vi "Climb Ramp.vi"(10 "Climb":bool, 11 "Plummet":bool) -> ()   [LabVIEW 2016]
uses:
  <vilib>/addons/control/pid/pid.llb/PID Control Input Filter (DBL).vi
  <vilib>/addons/control/pid/NI_PID_pid.lvlib
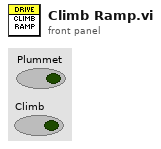
[diagram p1: front panel]
types:
  T1 = typedef "WPI_MotorControlDeviceRef.ctl" = cluster{"DeviceStatus":errorcluster, "Type":T2, "PWM":cluster{"PWM Channel":T3, "DeadBand":T4}, "CAN":cluster{"Device Number":u8, "SetOutput VI Ref":variant, "GetOutput VI Ref":variant, "Enable VI Ref":variant, "Disable VI Ref":variant, "Data":variant}, "Invert":bool}
  T2 = typedef "WPI_MotorControlType.ctl" = enum16{"PWM", "CAN"}
  T3 = typedef "FPGA_DIOPWMChannel.ctl" = enum8{"PWM 0", "PWM 1", "PWM 2", "PWM 3", "PWM 4", "PWM 5", "PWM 6", "PWM 7", "PWM 8", "PWM 9", "PWM MXP 0", "PWM MXP 1", "PWM MXP 2", "PWM MXP 3", "PWM MXP 4", "PWM MXP 5", "PWM MXP 6", "PWM MXP 7", "PWM MXP 8", "PWM MXP 9", "Invalid"}
  T4 = typedef "WPI_PWMDeadband.ctl" = cluster{"Name":string, "maxPositivePwm":i32, "minPositivePwm":i32, "centerPwm":i32, "maxNegativePwm":i32, "minNegativePwm":i32, "angularRange":u16}
  T5 = typedef "WPI_CANTalonSRX_GlobalStatus.ctl" = cluster{"Applied Throttle":dbl, "Module Enabled":bool, "CAN Error":errorcluster, "Closed Loop Error":dbl, "Forward Limit Switch Closed":bool, "Reverse Limit Switch Closed":bool, "Sensor Position":dbl, "Sensor Velocity":dbl, "Current":dbl, "Sticky Fault - Over Temp":bool, "Sticky Fault - Under Voltage":bool, "Sticky Fault - Forward Limit":bool, "Sticky Fault - Reverse Limit":bool, "Sticky Fault - Forward Soft Limit":bool, "Sticky Fault - Reverse Soft Limit":bool, "Brake is Enabled":bool, "Encoder Position":dbl, "Encoder Velocity":dbl, "Encoder Index Count":dbl, "Encoder A Pin State":bool, "Encoder B Pin State":bool, "Encoder Index Pin State":bool, "Analog In":dbl, "Analog In Velocity":dbl, "Temperature (C)":dbl, "Battery Voltage":dbl, "Control 5 Is Supported":bool, "Current Profile Slot Select":dbl, "Pos Div 8":bool, "Vel Div 4":bool, "Pulse Width Position":i32, "Pulse Width Velocity":i32, "Pulse Width Rise To Rise (us)":i32, "Pulse Width Rise To Fall (us)":i32, "Mot Prof Active Is Under Run":bool, "Mot Prof Active Has Under Run":bool, "Mot Prof Active Is Last":bool, "Mot Prof Active Velocity Only":bool, "Mot Prof Active Is Valid":bool, "Mot Prof Buffer Is Full":bool, "Mot Prof Active Profile Slot Select":i32, "Mot Prof NextID":i32, "Mot Prof Count":i32, "Mot Prof Active Velocity":dbl, "Mot Prof Active Position":dbl, "Mot Prof Output Enable":i32}
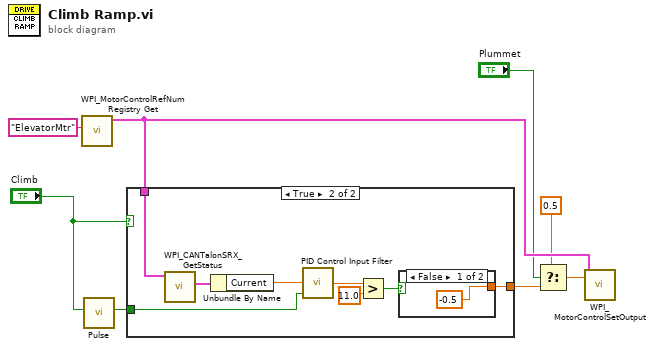
[diagram p0: block diagram]
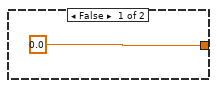
[diagram p2: hidden frame]
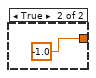
[diagram p3: hidden frame]
diagram:
  n1 = call <vilib>:"WPI_MotorControlRefNum Registry Get.vi"("refnum name"="ElevatorMtr") -> ("MotorControlDevRef"=w7:T1)  [unwired: 9 in, 1 out]
  n2 = call "Pulse.vi"("Input"="Climb") -> ("Output"=w2:bool)  [unwired: 10 in]
  n3 = case shown="True" "Climb" {
    tunnel: w7 -> [_ w16]
    tunnel: [0.0 w12] -> w6
    tunnel: w2 -> [_ w10]
    frame False {
    }
    frame True {
      n4 = call <vilib>:"WPI_CANTalonSRX_GetStatus.vi"("CAN Talon SRX Ref"=w16) -> ("Talon SRX Status"=w17:T5)  [unwired: 8 in, 2 out]
      n5 = Unbundle By Name(w17) -> ("Current"=w14:dbl)
      n6 = call-poly <vilib>:"PID Control Input Filter.vi"("reinitialize? (F)"=w10, "input"=w14) -> ("output"=w11:dbl)  [unwired: 3 in]
      n7 = Greater?(x=w11, y=11.0) -> (0:w15:bool)
      n8 = case shown="False" w15 {
        tunnel: [-0.5 -1.0] -> w12
        frame False {
        }
        frame True {
        }
      }
    }
  }
  n9 = Select(t=0.5, s="Plummet", f=w6) -> (s? t:f=w5:dbl)
  n10 = call <vilib>:"WPI_MotorControlSetOutput.vi"("Output"=w5, "MotorControlDevRef"=w7) -> ()  [unwired: 7 in, 3 out]
